vi "MU Calibration delete Analyze Result.vi"(8 "error in (no error)":errorcluster, 11 "analyzeResult":T1) -> (0 "error out":errorcluster)   [LabVIEW 2017, in "MU_3SL_interface.lvlib"]
doc: "MU_PUBLIC void MU_Calibration_deleteAnalyzeResult(\n MU_CalibrationAnalyzeResult* analyzeResult);"
uses:
  MU_3SL_interface.lvlib
  handles/CalibrationAnalyzeResultHandle.ctl
  lib/MU_3SL_interface.dll
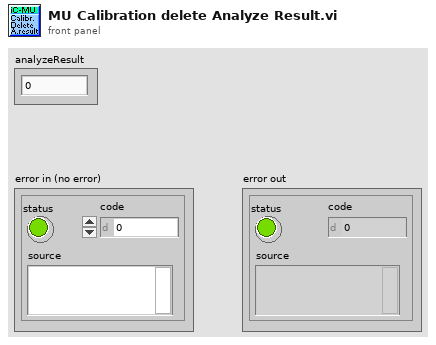
[diagram p1: front panel]
types:
  T1 = typedef "MU_3SL_interface.lvlib/CalibrationAnalyzeResultHandle.ctl" = u64
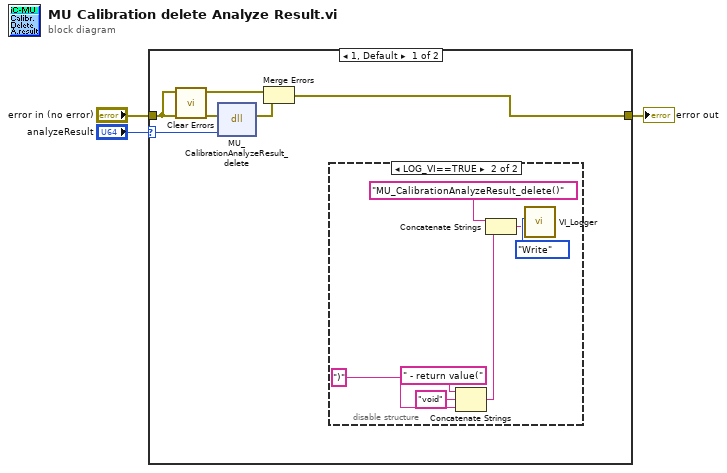
[diagram p0: block diagram]
diagram:
  n1 = case shown="1, Default" "analyzeResult" {
    selector: "analyzeResult" -> [w8 _]
    tunnel: "error in (no error)" -> [w6 w16]
    tunnel: [w4 w16] -> w1
    frame 1, Default {
      n2 = call <vilib>:"Clear Errors.vi"("error in (no error)"=w6) -> ("error out"=w7:errorcluster)  [unwired: 5 in, 1 out]
      n3 = dll-call lib="C:/Users/bes/AppData/Roaming/work/mu_9so/icsubmodules/soft_mu_3sl_master/lv_interface/lib/MU_3SL_interface**.*" fn="MU_CalibrationAnalyzeResult_delete"(error in=w7, "analyzeResult"=w8) -> (error out=w5:errorcluster)  [unwired: 4 in, 1 out]
      n4 = Merge Errors(w6, w5) -> (w4:errorcluster)
      n5 = disable-structure shown="LOG_VI==TRUE" {
        frame condition #0 {
        }
        frame condition #1 (active) {
          n6 = Concatenate Strings(" - return value(" ("string"), "void" ("string"), ")" ("string")) -> (w13:string)
          n7 = Concatenate Strings("MU_CalibrationAnalyzeResult_delete()" ("Info in"), w13) -> (w12:string)
          n8 = call "VI_Logger.vi"("Action (Read)"=enum16{"Write", "Read"}."Write", "Info in"=w12) -> ()  [unwired: 8 in, 2 out]
        }
      }
    }
    frame 0 {
    }
  }
  "error out" <- w1
